vi "加标模块单控对话框.vi"(11 "标题":string="加标模块") -> ()   [LabVIEW 2016, in "质控单元.lvlib"]
uses:
  <vilib>/Utility/miscctls.llb/LVPointTypeDef.ctl
panel:
  in  "柱塞泵调试":bool
  in  "流程参数读写":bool
  in  "定量":bool
  in  "排液":bool
  in  "退出":bool
  in  "搅拌":bool
  in  "进样":bool
  in  "停止":bool
  # "手动控制"
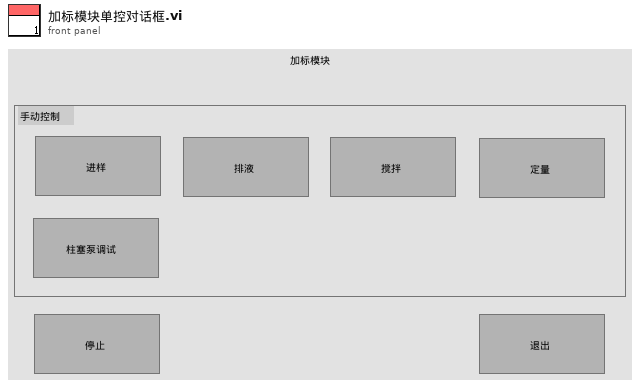
[diagram p1: front panel]
types:
  T1 = typedef "LVPointTypeDef.ctl" = cluster{"Horizontal":i16, "Vertical":i16}
  T2 = cluster{"氨氮":u8, "总磷":u8, "总氮":u8, "CODMn":u8, "CODCr":u8}
  T3 = enum16{"进样", "进样停止", "排液", "排液停止", "搅拌", "搅拌停止", "定量", "定量停止"}
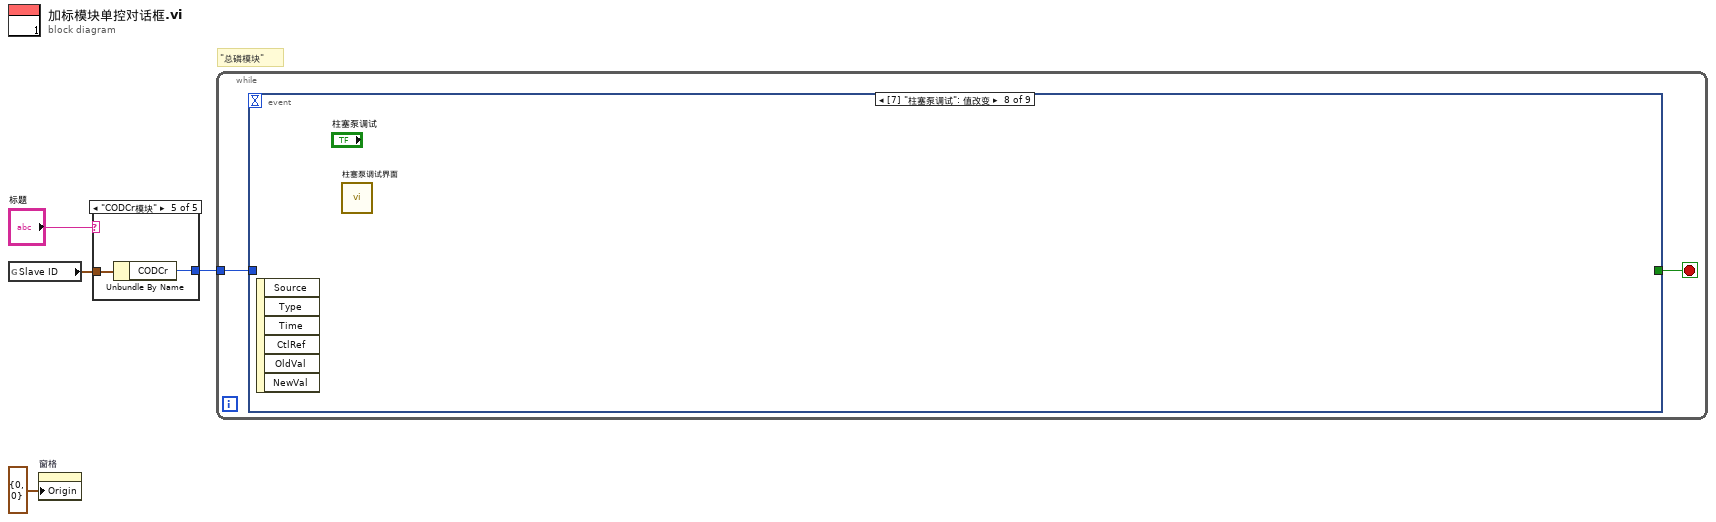
[diagram p0: block diagram]
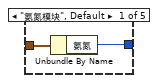
[diagram p2: hidden frame]
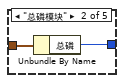
[diagram p3: hidden frame]
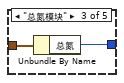
[diagram p4: hidden frame]
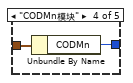
[diagram p5: hidden frame]
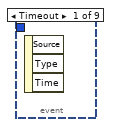
[diagram p6: hidden frame]
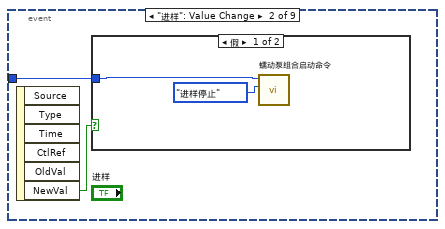
[diagram p7: hidden frame]
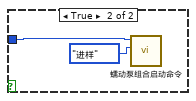
[diagram p8: hidden frame]
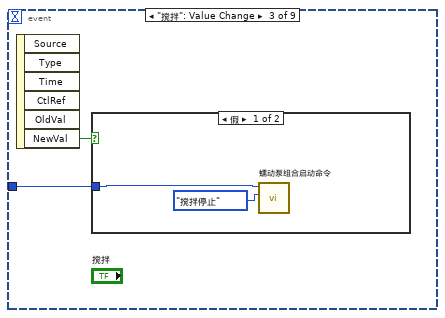
[diagram p9: hidden frame]
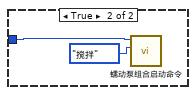
[diagram p10: hidden frame]
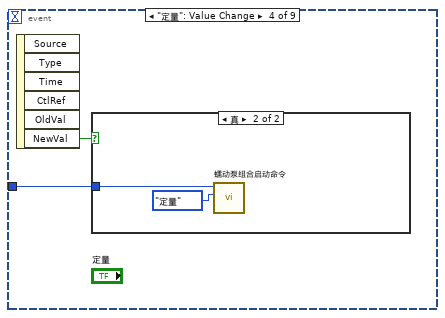
[diagram p11: hidden frame]
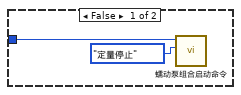
[diagram p12: hidden frame]
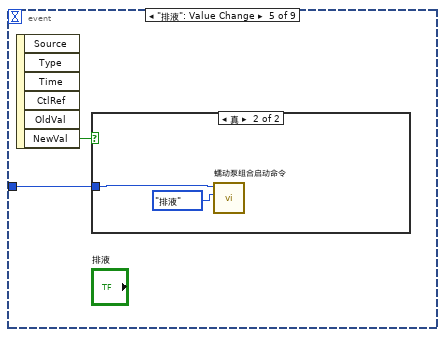
[diagram p13: hidden frame]
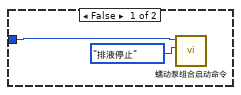
[diagram p14: hidden frame]
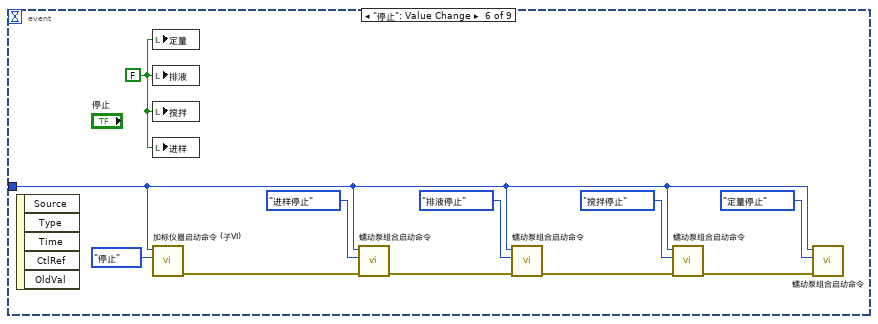
[diagram p15: hidden frame]
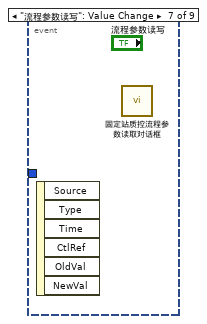
[diagram p16: hidden frame]
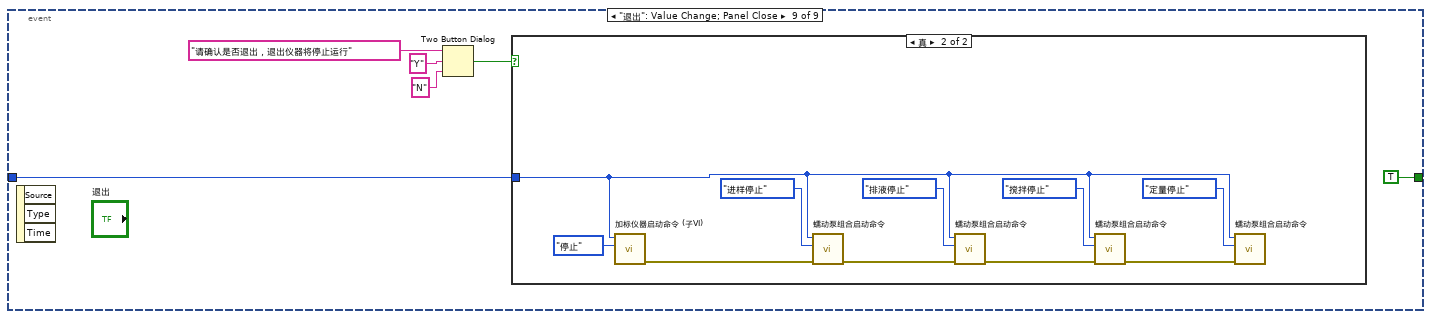
[diagram p17: hidden frame]
diagram:
  # "\"总磷模块\""
  n1 = global read "断电保存全局.vi" "Slave ID"() -> (w3:T2)
  n2 = property on="窗格" class="Pane"("Origin"=T1 {"Horizontal"=0, "Vertical"=0} ("原点")) -> ()  [unwired: 2 in, 2 out]
  n3 = case shown="\"CODCr模块\"" "标题" {
    tunnel: [w5 w7 w9 w11 w13] -> w1
    tunnel: w3 -> [w6 w8 w10 w12 w14]
    frame "氨氮模块", Default {
      n4 = Unbundle By Name(w6) -> ("氨氮"=w5:u8)
    }
    frame "总磷模块" {
      n5 = Unbundle By Name(w8) -> ("总磷"=w7:u8)
    }
    frame "总氮模块" {
      n6 = Unbundle By Name(w10) -> ("总氮"=w9:u8)
    }
    frame "CODMn模块" {
      n7 = Unbundle By Name(w12) -> ("CODMn"=w11:u8)
    }
    frame "CODCr模块" {
      n8 = Unbundle By Name(w14) -> ("CODCr"=w13:u8)
    }
  }
  n9 = while {
    tunnel: w1 -> [w15]
    stop <- w16 stop-if-true
    n10 = event shown="[7] \"柱塞泵调试\": 值改变" {
      selector: _ -> [_ _ _ _ _ _ _ _ _]
      dyn-events: _ -> [_ _ _ _ _ _ _ _ _]
      timeout: _ -> [_ _ _ _ _ _ _ _ _]
      tunnel: [_ _ _ _ _ _ _ _ TRUE] -> w16
      tunnel: w15 -> [_ w17 w23 w29 w35 w41 _ _ w52]
      event Timeout {
        n11 = event-data() -> ()  [unwired: 1 in, 3 out]
      }
      event "进样": Value Change {
        n12 = event-data() -> ("NewVal"=w18:bool)  [unwired: 1 in, 5 out]
        n13 = case shown="假" w18 {
          tunnel: w17 -> [w19 w22]
          frame False {
            n14 = call "蠕动泵组合启动命令.vi"("控制方式"=T3."进样停止", "仪器"=w19) -> ()  [unwired: 9 in, 1 out]
          }
          frame True {
            n15 = call "蠕动泵组合启动命令.vi"("控制方式"=T3."进样", "仪器"=w22) -> ()  [unwired: 9 in, 1 out]
          }
        }
      }
      event "搅拌": Value Change {
        n16 = event-data() -> ("NewVal"=w24:bool)  [unwired: 1 in, 5 out]
        n17 = case shown="假" w24 {
          tunnel: w23 -> [w25 w28]
          frame False {
            n18 = call "蠕动泵组合启动命令.vi"("控制方式"=T3."搅拌停止", "仪器"=w25) -> ()  [unwired: 9 in, 1 out]
          }
          frame True {
            n19 = call "蠕动泵组合启动命令.vi"("控制方式"=T3."搅拌", "仪器"=w28) -> ()  [unwired: 9 in, 1 out]
          }
        }
      }
      event "定量": Value Change {
        n20 = event-data() -> ("NewVal"=w30:bool)  [unwired: 1 in, 5 out]
        n21 = case shown="真" w30 {
          tunnel: w29 -> [w31 w34]
          frame False {
            n22 = call "蠕动泵组合启动命令.vi"("控制方式"=T3."定量停止", "仪器"=w31) -> ()  [unwired: 9 in, 1 out]
          }
          frame True {
            n23 = call "蠕动泵组合启动命令.vi"("控制方式"=T3."定量", "仪器"=w34) -> ()  [unwired: 9 in, 1 out]
          }
        }
      }
      event "排液": Value Change {
        n24 = event-data() -> ("NewVal"=w36:bool)  [unwired: 1 in, 5 out]
        n25 = case shown="真" w36 {
          tunnel: w35 -> [w37 w40]
          frame False {
            n26 = call "蠕动泵组合启动命令.vi"("控制方式"=T3."排液停止", "仪器"=w37) -> ()  [unwired: 9 in, 1 out]
          }
          frame True {
            n27 = call "蠕动泵组合启动命令.vi"("控制方式"=T3."排液", "仪器"=w40) -> ()  [unwired: 9 in, 1 out]
          }
        }
      }
      event "停止": Value Change {
        w42 = FALSE ("搅拌")
        n28 = event-data() -> ()  [unwired: 1 in, 5 out]
        n29 = local write "定量"(w42) -> ()
        n30 = local write "排液"(w42) -> ()
        n31 = local write "搅拌"(w42) -> ()
        n32 = local write "进样"(w42) -> ()
        n33 = call "加标仪器启动命令 (子VI).vi"("启动命令"=enum16{"启动水样流程", "启动加标流程", "排液", "停止"}."停止", "仪器"=w41) -> ("错误输出"=w46:errorcluster)  [unwired: 9 in]
        n34 = call "蠕动泵组合启动命令.vi"("Error in"=w46, "控制方式"=T3."进样停止", "仪器"=w41) -> ("error out"=w45:errorcluster)  [unwired: 8 in]
        n35 = call "蠕动泵组合启动命令.vi"("Error in"=w45, "控制方式"=T3."排液停止", "仪器"=w41) -> ("error out"=w44:errorcluster)  [unwired: 8 in]
        n36 = call "蠕动泵组合启动命令.vi"("Error in"=w44, "控制方式"=T3."搅拌停止", "仪器"=w41) -> ("error out"=w43:errorcluster)  [unwired: 8 in]
        n37 = call "蠕动泵组合启动命令.vi"("Error in"=w43, "控制方式"=T3."定量停止", "仪器"=w41) -> ()  [unwired: 8 in, 1 out]
      }
      event "流程参数读写": Value Change {
        n38 = event-data() -> ()  [unwired: 1 in, 6 out]
        n39 = call "固定站质控流程参数读取对话框.vi"() -> ()  [unwired: 12 in]
      }
      event "柱塞泵调试": Value Change {
        n40 = event-data() -> ()  [unwired: 1 in, 6 out]
        n41 = call "柱塞泵调试界面.vi"() -> ()  [unwired: 16 in]
      }
      event "退出": Value Change; Panel Close {
        n42 = event-data() -> ()  [unwired: 1 in, 3 out]
        n43 = Two Button Dialog(message="请确认是否退出，退出仪器将停止运行" ("消息"), 1:"N" ("F按钮名称（“取消”）"), 2:"Y" ("T按钮名称（“确定”）")) -> (T button?=w53:bool)
        n44 = case shown="真" w53 {
          tunnel: w52 -> [_ w58]
          frame False {
          }
          frame True {
            n45 = call "加标仪器启动命令 (子VI).vi"("启动命令"=enum16{"启动水样流程", "启动加标流程", "排液", "停止"}."停止", "仪器"=w58) -> ("错误输出"=w62:errorcluster)  [unwired: 9 in]
            n46 = call "蠕动泵组合启动命令.vi"("Error in"=w62, "控制方式"=T3."进样停止", "仪器"=w58) -> ("error out"=w61:errorcluster)  [unwired: 8 in]
            n47 = call "蠕动泵组合启动命令.vi"("Error in"=w61, "控制方式"=T3."排液停止", "仪器"=w58) -> ("error out"=w60:errorcluster)  [unwired: 8 in]
            n48 = call "蠕动泵组合启动命令.vi"("Error in"=w60, "控制方式"=T3."搅拌停止", "仪器"=w58) -> ("error out"=w59:errorcluster)  [unwired: 8 in]
            n49 = call "蠕动泵组合启动命令.vi"("Error in"=w59, "控制方式"=T3."定量停止", "仪器"=w58) -> ()  [unwired: 8 in, 1 out]
          }
        }
      }
    }
  }
